vi "Table Value To 1D DBL.vi"(11 "Table Ref In":refnum<vi>) -> (1 "DBL Out":dbl[](array[numeric]), 3 "Table Ref Out":refnum<vi>)   [LabVIEW 2024]
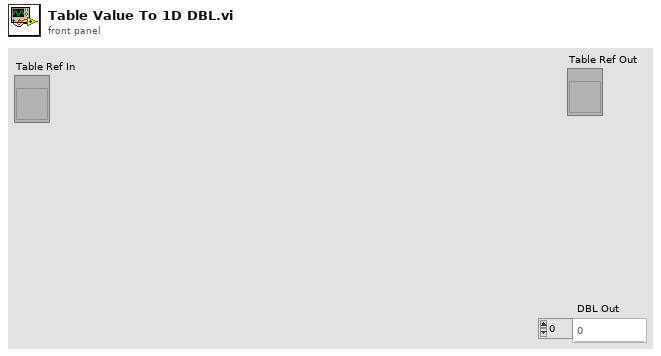
[diagram p1: front panel]
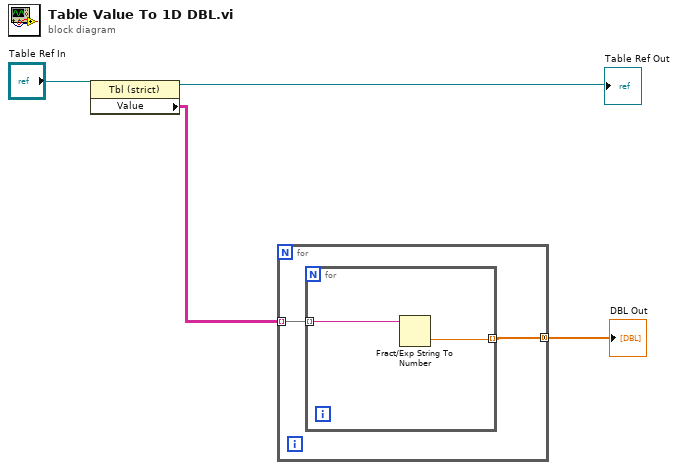
[diagram p0: block diagram]
diagram:
  n1 = property class="Tbl (strict)"(reference="Table Ref In") -> (reference out=→"Table Ref Out":refnum<vi>, "Value"=w2:string[][])  [unwired: 1 in, 1 out]
  n2 = for {
    tunnel: w2 -> [w6] mode=indexing
    tunnel: [w5] -> w1 mode=concatenating
    n3 = for {
      tunnel: w6 -> [w8] mode=indexing
      tunnel: [w7] -> w5 mode=indexing
      n4 = Fract/Exp String To Number(string=w8) -> (number=w7:dbl)  [unwired: 3 in, 1 out]
    }
  }
  "DBL Out" <- w1
